vi "ComparePositionToWaypoint.vi"(8 "Waypoint Index":dbl, 11 "distance (dm)":dbl) -> (0 "Next Waypoint Index":dbl, 3 "Close to Waypoint":bool)   [LabVIEW 2011]
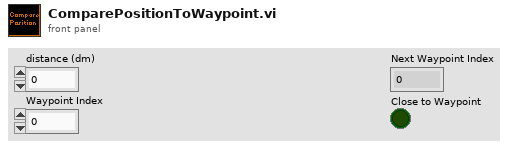
[diagram p1: front panel]
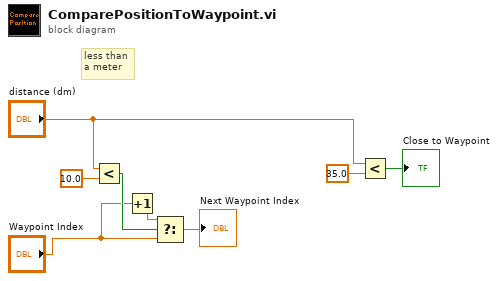
[diagram p0: block diagram]
diagram:
  # "less than \na meter"
  n1 = Less?(x="distance (dm)", y=10.0) -> (x < y?=w7:bool)
  n2 = Increment(x="Waypoint Index") -> (x+1=w6:dbl)
  n3 = Select(t=w6, s=w7, f="Waypoint Index") -> (s? t:f=→"Next Waypoint Index":dbl)
  n4 = Less?(x="distance (dm)", y=35.0) -> (x < y?=→"Close to Waypoint":bool)
